vi "Setup For Triggered Images USB3 v4.3.vi"(5 "error in":errorcluster caption="error in (no error)", 6 "Timeout":u32, 7 "Gain":dbl, 8 "Shutter speed":dbl=0.1, 9 "Camera Name":T3="cam0") -> (0 "Error out":errorcluster caption="error in (no error)", 1 "Session Out":T3="cam0", 2 "Height":u32, 3 "Width":u32, 4 "DeviceID":string)   [LabVIEW 2013]
doc: "The Grab and Attributes Setup VI acquires images continuously and displays the images in an image control using high-level acquisition VIs. The VI also modifes the camera attributes while acquiring images. A grab is appropriate for high-speed applications in which you need to process only one image at a time."
uses:
  <vilib>/userdefined/High Color/IMAQdx.ctl
  <vilib>/vision/driver/IMAQdx.llb/IMAQdx Attribute Type.ctl
  <vilib>/vision/driver/IMAQdx.llb/IMAQdx Attribute Visibility.ctl
  <vilib>/vision/driver/NI_Vision_Acquisition_Software.lvlib
  <resource>/objmgr/imaqdx.rc
panel:
  out "Attribute Information Array":T2(array[cluster])=[{"Attribute Type"=enum."DBL", "Readable"=TRUE, "Writable"=TRUE, "Attribute Name"="CameraAttributes::AnalogControl::Gain"}, {"Attribute Type"=enum."DBL", "Readable"=TRUE, "Writable"=TRUE, "Attribute Name"="CameraAttributes::AnalogControl::BlackLevel"}, {"Attribute Type"=enum."DBL", "Readable"=TRUE, "Writable"=FALSE, "Attribute Name"="CameraAttributes::AnalogControl::Gamma"}, {"Attribute Type"=enum."Bool", "Readable"=TRUE, "Writable"=TRUE, "Attribute Name"="CameraAttributes::AnalogControl::GammaEnabled"}, {"Attribute Type"=enum."I64", "Readable"=TRUE, "Writable"=FALSE, "Attribute Name"="CameraAttributes::AnalogControl::Sharpness"}, {"Attribute Type"=enum."String", "Readable"=TRUE, "Writable"=FALSE, "Attribute Name"="CameraAttributes::DeviceControl::DeviceVendorName"}, {"Attribute Type"=enum."String", "Readable"=TRUE, "Writable"=FALSE, "Attribute Name"="CameraAttributes::DeviceControl::DeviceModelName"}, {"Attribute Type"=enum."String", "Readable"=TRUE, "Writable"=FALSE, "Attribute Name"="CameraAttributes::DeviceControl::DeviceFamilyName"}, {"Attribute Type"=enum."String", "Readable"=TRUE, "Writable"=FALSE, "Attribute Name"="CameraAttributes::DeviceControl::DeviceVersion"}, {"Attribute Type"=enum."String", "Readable"=TRUE, "Writable"=FALSE, "Attribute Name"="CameraAttributes::DeviceControl::DeviceSVNVersion"}, {"Attribute Type"=enum."String", "Readable"=TRUE, "Writable"=FALSE, "Attribute Name"="CameraAttributes::DeviceControl::DeviceID"}, {"Attribute Type"=enum."String", "Readable"=TRUE, "Writable"=TRUE, "Attribute Name"="CameraAttributes::DeviceControl::DeviceUserID"}, {"Attribute Type"=enum."Enum", "Readable"=TRUE, "Writable"=TRUE, "Attribute Name"="CameraAttributes::AcquisitionControl::TriggerSelector"}, {"Attribute Type"=enum."Enum", "Readable"=TRUE, "Writable"=TRUE, "Attribute Name"="CameraAttributes::AcquisitionControl::TriggerMode"}, {"Attribute Type"=enum."Command", "Readable"=FALSE, "Writable"=FALSE, "Attribute Name"="CameraAttributes::AcquisitionControl::TriggerSoftware"}, {"Attribute Type"=enum."Enum", "Readable"=TRUE, "Writable"=TRUE, "Attribute Name"="CameraAttributes::AcquisitionControl::TriggerSource"}, {"Attribute Type"=enum."Enum", "Readable"=TRUE, "Writable"=TRUE, "Attribute Name"="CameraAttributes::AcquisitionControl::TriggerActivation"}, {"Attribute Type"=enum."Enum", "Readable"=TRUE, "Writable"=TRUE, "Attribute Name"="CameraAttributes::AcquisitionControl::ExposureMode"}, {"Attribute Type"=enum."Enum", "Readable"=FALSE, "Writable"=FALSE, "Attribute Name"="CameraAttributes::AcquisitionControl::ExposureAuto"}, {"Attribute Type"=enum."DBL", "Readable"=TRUE, "Writable"=FALSE, "Attribute Name"="CameraAttributes::AcquisitionControl::ExposureTime"}, {"Attribute Type"=enum."Enum", "Readable"=TRUE, "Writable"=TRUE, "Attribute Name"="CameraAttributes::AcquisitionControl::AcquisitionMode"}, {"Attribute Type"=enum."Enum", "Readable"=TRUE, "Writable"=FALSE, "Attribute Name"="CameraAttributes::AcquisitionControl::AcquisitionFrameRateAuto"}, {"Attribute Type"=enum."Bool", "Readable"=FALSE, "Writable"=FALSE, "Attribute Name"="CameraAttributes::AcquisitionControl::AcquisitionFrameRateEnabled"}, {"Attribute Type"=enum."DBL", "Readable"=FALSE, "Writable"=FALSE, "Attribute Name"="CameraAttributes::AcquisitionControl::AcquisitionFrameRate"}, {"Attribute Type"=enum."I64", "Readable"=FALSE, "Writable"=FALSE, "Attribute Name"="CameraAttributes::AcquisitionControl::AcquisitionFrameCount"}, {"Attribute Type"=enum."Enum", "Readable"=TRUE, "Writable"=TRUE, "Attribute Name"="CameraAttributes::ImageFormatControl::PixelFormat"}, {"Attribute Type"=enum."I64", "Readable"=TRUE, "Writable"=TRUE, "Attribute Name"="CameraAttributes::ImageFormatControl::Width"}, {"Attribute Type"=enum."I64", "Readable"=TRUE, "Writable"=TRUE, "Attribute Name"="CameraAttributes::ImageFormatControl::Height"}, {"Attribute Type"=enum."I64", "Readable"=TRUE, "Writable"=TRUE, "Attribute Name"="CameraAttributes::ImageFormatControl::OffsetX"}, {"Attribute Type"=enum."I64", "Readable"=TRUE, "Writable"=TRUE, "Attribute Name"="CameraAttributes::ImageFormatControl::OffsetY"}, {"Attribute Type"=enum."Enum", "Readable"=TRUE, "Writable"=FALSE, "Attribute Name"="CameraAttributes::ImageFormatControl::PixelCoding"}, {"Attribute Type"=enum."I64", "Readable"=TRUE, "Writable"=FALSE, "Attribute Name"="CameraAttributes::ImageFormatControl::PixelDynamicRangeMin"}, {"Attribute Type"=enum."I64", "Readable"=TRUE, "Writable"=FALSE, "Attribute Name"="CameraAttributes::ImageFormatControl::PixelDynamicRangeMax"}, {"Attribute Type"=enum."Enum", "Readable"=TRUE, "Writable"=TRUE, "Attribute Name"="CameraAttributes::ImageFormatControl::TestImageSelector"}, {"Attribute Type"=enum."I64", "Readable"=TRUE, "Writable"=FALSE, "Attribute Name"="CameraAttributes::UserSetControl::UserSetCurrent"}, {"Attribute Type"=enum."Enum", "Readable"=TRUE, "Writable"=TRUE, "Attribute Name"="CameraAttributes::UserSetControl::UserSetSelector"}, {"Attribute Type"=enum."Command", "Readable"=FALSE, "Writable"=TRUE, "Attribute Name"="CameraAttributes::UserSetControl::UserSetLoad"}, {"Attribute Type"=enum."Command", "Readable"=FALSE, "Writable"=TRUE, "Attribute Name"="CameraAttributes::UserSetControl::UserSetSave"}, {"Attribute Type"=enum."DBL", "Readable"=FALSE, "Writable"=FALSE, "Attribute Name"="CameraAttributes::DigitalIOControl::StrobeDelay"}, {"Attribute Type"=enum."DBL", "Readable"=FALSE, "Writable"=FALSE, "Attribute Name"="CameraAttributes::DigitalIOControl::StrobeDuration"}]
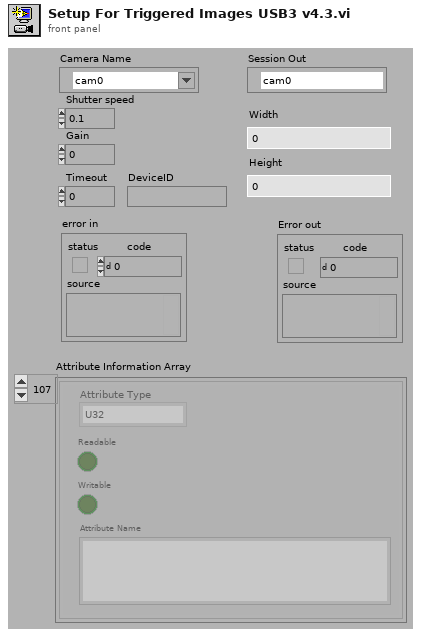
[diagram p1: front panel]
types:
  T1 = typedef "NI_Vision_Acquisition_Software.lvlib/IMAQdx Attribute Type.ctl" = enum32{"U32", "I64", "DBL", "String", "Enum", "Bool", "Command"}
  T2 = cluster{"Attribute Type":T1, "Readable":bool, "Writable":bool, "Attribute Name":string}[]
  T3 = typedef "IMAQdx.ctl" = refnum<k21>
  T4 = typedef "NI_Vision_Acquisition_Software.lvlib/IMAQdx Attribute Visibility.ctl" = enum32{"Simple", "Intermediate", "Advanced"}
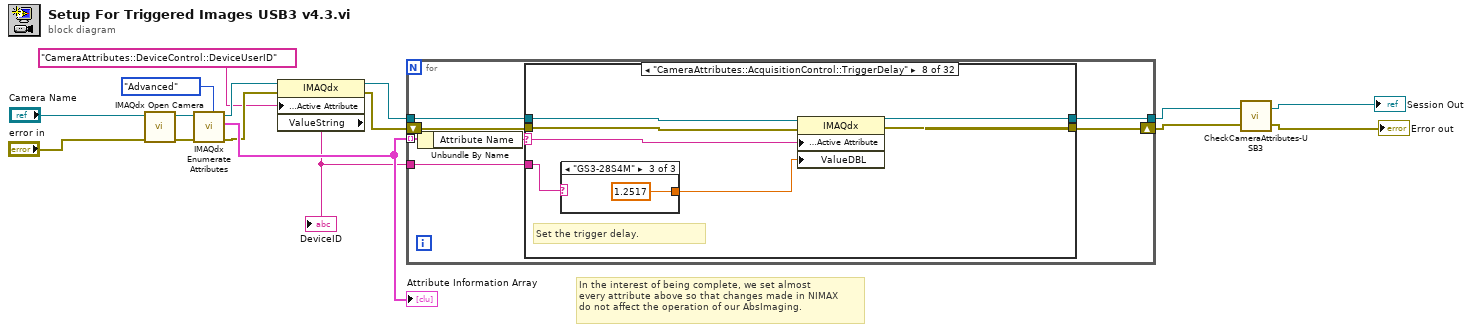
[diagram p0: block diagram]
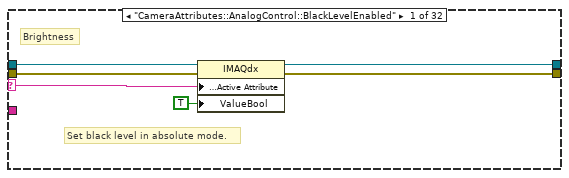
[diagram p2: hidden frame]
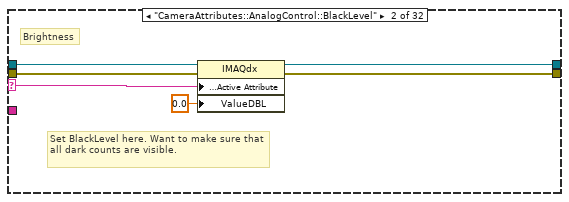
[diagram p3: hidden frame]
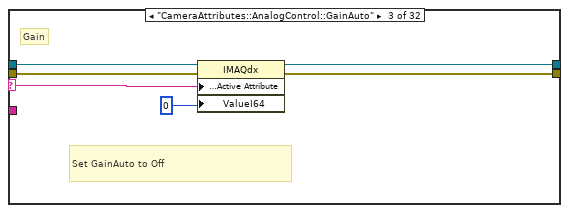
[diagram p4: hidden frame]
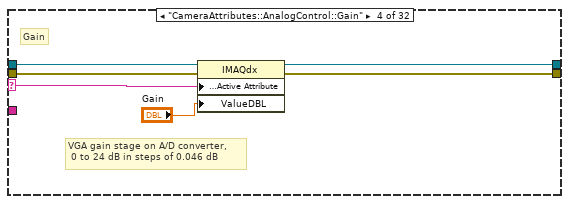
[diagram p5: hidden frame]
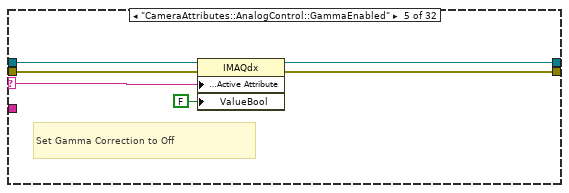
[diagram p6: hidden frame]
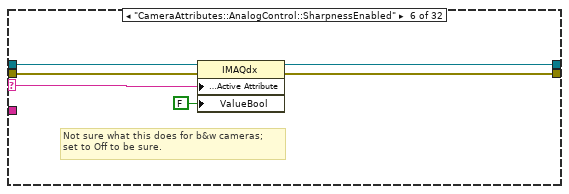
[diagram p7: hidden frame]
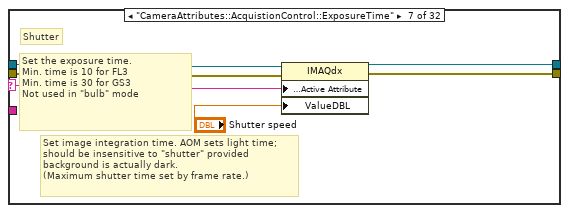
[diagram p8: hidden frame]
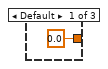
[diagram p9: hidden frame]
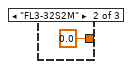
[diagram p10: hidden frame]
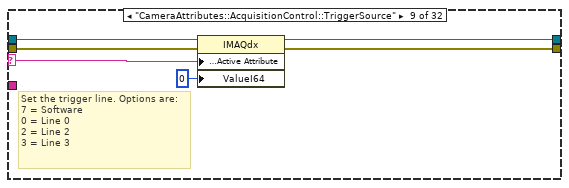
[diagram p11: hidden frame]
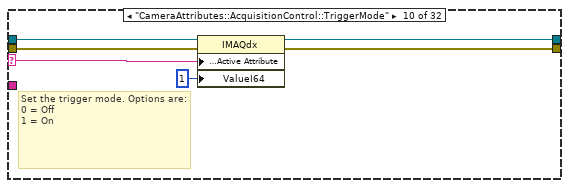
[diagram p12: hidden frame]
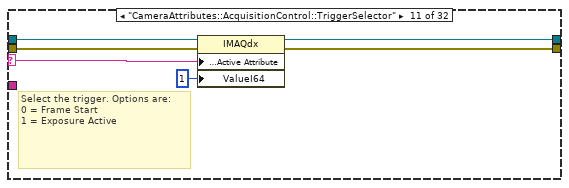
[diagram p13: hidden frame]
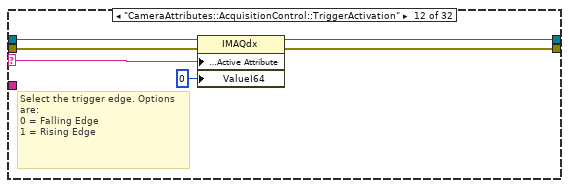
[diagram p14: hidden frame]
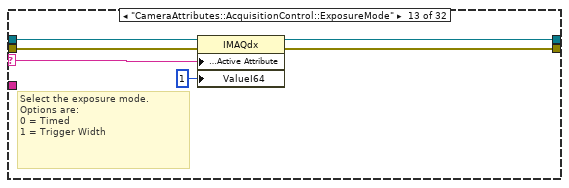
[diagram p15: hidden frame]
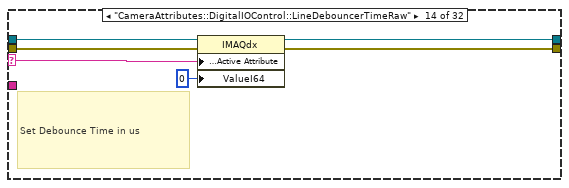
[diagram p16: hidden frame]
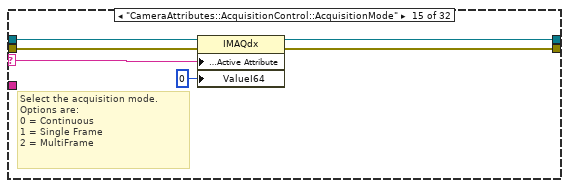
[diagram p17: hidden frame]
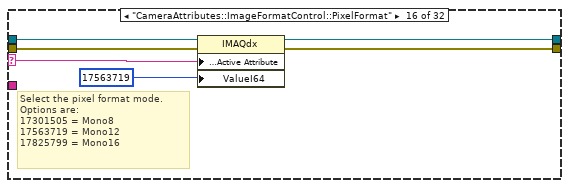
[diagram p18: hidden frame]
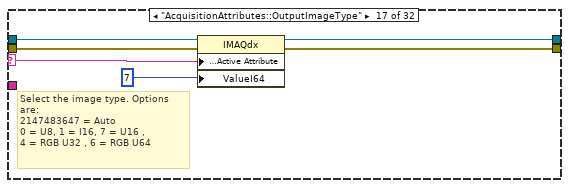
[diagram p19: hidden frame]
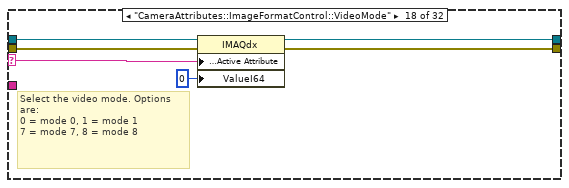
[diagram p20: hidden frame]
diagram:
  # "In the interest of being complete, we set almost\nevery attribute above so that changes made in NIMAX\ndo not affect the operation of our AbsImaging."
  n1 = call <vilib>:"IMAQdx Open Camera.vi"("error in"="error in", "Session In"="Camera Name") -> ("error out"=w14:errorcluster, "Session Out"=w15:T3)  [unwired: 1 in, 7 out]
  n2 = call <vilib>:"IMAQdx Enumerate Attributes.vi"("Visibility"=IMAQdx_Attribute_Visibility."Advanced", "error in"=w14, "Session In"=w15) -> ("error out"=w9:errorcluster, "Attribute Information Array"=w11:T2, "Session Out"=w10:T3)  [unwired: 1 in, 5 out]
  "Attribute Information Array" <- w11
  n3 = property class="IMAQdx"(reference=w10, error in=w9, "Camera Attributes:Active Attribute"="CameraAttributes::DeviceControl::DeviceUserID" ("ActiveAttribute")) -> (reference out=w7:T3, error out=w8:errorcluster, "ValueString"=w6:string)
  "DeviceID" <- w6
  n4 = for {
    tunnel: w11 -> [w23] mode=indexing
    tunnel: w7 -> [w18]
    tunnel: [w21] -> w3
    shift-right: [w20] -> w4
    shift-left: w8 -> [w19]
    tunnel: w6 -> [w17]
    n5 = Unbundle By Name(w23) -> ("Attribute Name"=w22:string)
    n6 = case shown="\"CameraAttributes::AcquisitionControl::TriggerDelay\"" w22 {
      selector: w22 -> [w25 w31 w37 w43 w49 w55 w61 w68 w77 w83 w89 w95 w101 w107 w113 w119 w125 w131 w137 w143 w151 w161 w170 w176 w182 w188 w194 w199 w205 w211 w217 _]
      tunnel: w18 -> [w29 w35 w41 w47 w53 w59 w65 w72 w81 w87 w93 w99 w105 w111 w117 w123 w129 w135 w141 w147 w150 w160 w169 w175 w181 w187 w193 w203 w209 w215 w221 w223]
      tunnel: w19 -> [w28 w34 w40 w46 w52 w58 w64 w71 w80 w86 w92 w98 w104 w110 w116 w122 w128 w134 w140 w146 w154 w164 w173 w179 w185 w191 w197 w202 w208 w214 w220 w222]
      tunnel: [w27 w33 w39 w45 w51 w57 w63 w70 w79 w85 w91 w97 w103 w109 w115 w121 w127 w133 w139 w145 w153 w163 w172 w178 w184 w190 w196 w201 w207 w213 w219 w223] -> w21
      tunnel: [w26 w32 w38 w44 w50 w56 w62 w69 w78 w84 w90 w96 w102 w108 w114 w120 w126 w132 w138 w144 w152 w162 w171 w177 w183 w189 w195 w200 w206 w212 w218 w222] -> w20
      tunnel: w17 -> [_ _ _ _ _ _ _ w67 _ _ _ _ _ _ _ _ _ _ _ _ w149 w159 _ _ _ _ _ _ _ _ _ _]
      frame "CameraAttributes::AnalogControl::BlackLevelEnabled" {
        # "Set black level in absolute mode."
        # "Brightness"
        n7 = property class="IMAQdx"(reference=w29, error in=w28, "Camera Attributes:Active Attribute"=w25, "ValueBool"=TRUE) -> (reference out=w27:T3, error out=w26:errorcluster)
      }
      frame "CameraAttributes::AnalogControl::BlackLevel" {
        # "Set BlackLevel here. Want to make sure that all dark counts are visible."
        # "Brightness"
        n8 = property class="IMAQdx"(reference=w35, error in=w34, "Camera Attributes:Active Attribute"=w31, "ValueDBL"=0.0) -> (reference out=w33:T3, error out=w32:errorcluster)
      }
      frame "CameraAttributes::AnalogControl::GainAuto" {
        # "Set GainAuto to Off"
        # "Gain"
        n9 = property class="IMAQdx"(reference=w41, error in=w40, "Camera Attributes:Active Attribute"=w37, "ValueI64"=i64 0) -> (reference out=w39:T3, error out=w38:errorcluster)
      }
      frame "CameraAttributes::AnalogControl::Gain" {
        # "VGA gain stage on A/D converter,\n 0 to 24 dB in steps of 0.046 dB"
        # "Gain"
        n10 = property class="IMAQdx"(reference=w47, error in=w46, "Camera Attributes:Active Attribute"=w43, "ValueDBL"="Gain") -> (reference out=w45:T3, error out=w44:errorcluster)
      }
      frame "CameraAttributes::AnalogControl::GammaEnabled" {
        # "Set Gamma Correction to Off"
        n11 = property class="IMAQdx"(reference=w53, error in=w52, "Camera Attributes:Active Attribute"=w49, "ValueBool"=FALSE) -> (reference out=w51:T3, error out=w50:errorcluster)
      }
      frame "CameraAttributes::AnalogControl::SharpnessEnabled" {
        # "Not sure what this does for b&w cameras;\nset to Off to be sure."
        n12 = property class="IMAQdx"(reference=w59, error in=w58, "Camera Attributes:Active Attribute"=w55, "ValueBool"=FALSE) -> (reference out=w57:T3, error out=w56:errorcluster)
      }
      frame "CameraAttributes::AcquistionControl::ExposureTime" {
        # "Set the exposure time.\nMin. time is 10 for FL3\nMin. time is 30 for GS3\nNot used in \"bulb\" mode"
        # "Set image integration time. AOM sets light time;\nshould be insensitive to \"shutter\" provided \nbackground is actually dark.\n(Maximum shutter time set by frame rate.)"
        # "Shutter"
        n13 = property class="IMAQdx"(reference=w65, error in=w64, "Camera Attributes:Active Attribute"=w61, "ValueDBL"="Shutter speed") -> (reference out=w63:T3, error out=w62:errorcluster)
      }
      frame "CameraAttributes::AcquisitionControl::TriggerDelay" {
        # "Set the trigger delay."
        n14 = case shown="\"GS3-28S4M\"" w67 {
          tunnel: [0.0 ("ValueDBL") 0.0 ("ValueDBL") 1.2517 ("ValueDBL")] -> w66
          frame Default {
          }
          frame "FL3-32S2M" {
          }
          frame "GS3-28S4M" {
          }
        }
        n15 = property class="IMAQdx"(reference=w72, error in=w71, "Camera Attributes:Active Attribute"=w68, "ValueDBL"=w66) -> (reference out=w70:T3, error out=w69:errorcluster)
      }
      frame "CameraAttributes::AcquisitionControl::TriggerSource" {
        # "Set the trigger line. Options are:\n7 = Software\n0 = Line 0\n2 = Line 2\n3 = Line 3"
        n16 = property class="IMAQdx"(reference=w81, error in=w80, "Camera Attributes:Active Attribute"=w77, "ValueI64"=i64 0) -> (reference out=w79:T3, error out=w78:errorcluster)
      }
      frame "CameraAttributes::AcquisitionControl::TriggerMode" {
        # "Set the trigger mode. Options are:\n0 = Off\n1 = On"
        n17 = property class="IMAQdx"(reference=w87, error in=w86, "Camera Attributes:Active Attribute"=w83, "ValueI64"=i64 1) -> (reference out=w85:T3, error out=w84:errorcluster)
      }
      frame "CameraAttributes::AcquisitionControl::TriggerSelector" {
        # "Select the trigger. Options are:\n0 = Frame Start\n1 = Exposure Active"
        n18 = property class="IMAQdx"(reference=w93, error in=w92, "Camera Attributes:Active Attribute"=w89, "ValueI64"=i64 1) -> (reference out=w91:T3, error out=w90:errorcluster)
      }
      frame "CameraAttributes::AcquisitionControl::TriggerActivation" {
        # "Select the trigger edge. Options are:\n0 = Falling Edge\n1 = Rising Edge"
        n19 = property class="IMAQdx"(reference=w99, error in=w98, "Camera Attributes:Active Attribute"=w95, "ValueI64"=i64 0) -> (reference out=w97:T3, error out=w96:errorcluster)
      }
      frame "CameraAttributes::AcquisitionControl::ExposureMode" {
        # "Select the exposure mode. Options are:\n0 = Timed\n1 = Trigger Width"
        n20 = property class="IMAQdx"(reference=w105, error in=w104, "Camera Attributes:Active Attribute"=w101, "ValueI64"=i64 1) -> (reference out=w103:T3, error out=w102:errorcluster)
      }
      frame "CameraAttributes::DigitalIOControl::LineDebouncerTimeRaw" {
        # "Set Debounce Time in us"
        n21 = property class="IMAQdx"(reference=w111, error in=w110, "Camera Attributes:Active Attribute"=w107, "ValueI64"=i64 0) -> (reference out=w109:T3, error out=w108:errorcluster)
      }
      frame "CameraAttributes::AcquisitionControl::AcquisitionMode" {
        # "Select the acquisition mode. Options are:\n0 = Continuous\n1 = Single Frame\n2 = MultiFrame"
        n22 = property class="IMAQdx"(reference=w117, error in=w116, "Camera Attributes:Active Attribute"=w113, "ValueI64"=i64 0) -> (reference out=w115:T3, error out=w114:errorcluster)
      }
      frame "CameraAttributes::ImageFormatControl::PixelFormat" {
        # "Select the pixel format mode. Options are:\n17301505 = Mono8\n17563719 = Mono12\n17825799 = Mono16"
        n23 = property class="IMAQdx"(reference=w123, error in=w122, "Camera Attributes:Active Attribute"=w119, "ValueI64"=i64 17563719) -> (reference out=w121:T3, error out=w120:errorcluster)
      }
      frame "AcquisitionAttributes::OutputImageType" {
        # "Select the image type. Options are:\n2147483647 = Auto\n0 = U8, 1 = I16, 7 = U16 , \n4 = RGB U32 , 6 = RGB U64"
        n24 = property class="IMAQdx"(reference=w129, error in=w128, "Camera Attributes:Active Attribute"=w125, "ValueI64"=i64 7) -> (reference out=w127:T3, error out=w126:errorcluster)
      }
      frame "CameraAttributes::ImageFormatControl::VideoMode" {
        # "Select the video mode. Options are:\n0 = mode 0, 1 = mode 1\n7 = mode 7, 8 = mode 8"
        n25 = property class="IMAQdx"(reference=w135, error in=w134, "Camera Attributes:Active Attribute"=w131, "ValueI64"=i64 0) -> (reference out=w133:T3, error out=w132:errorcluster)
      }
      frame "CameraAttributes::AcquisitionControl::pgrExposureCompensationAuto" {
        # "Select the exposure compensation mode. Options are:\n0 = off, 2 = continuous"
        n26 = property class="IMAQdx"(reference=w141, error in=w140, "Camera Attributes:Active Attribute"=w137, "ValueU32"=u32 0) -> (reference out=w139:T3, error out=w138:errorcluster)
      }
      frame "CameraAttributes::AcquisitionControl::pgrExposureCompensation" {
        # "Select the exposure compensation in EV\n\n0.001 gives zero"
        n27 = property class="IMAQdx"(reference=w147, error in=w146, "Camera Attributes:Active Attribute"=w143, "ValueDBL"=0.001) -> (reference out=w145:T3, error out=w144:errorcluster)
      }
      frame "CameraAttributes::ImageFormatControl::Width" {
        # "Select the width. Max is 2080 for FL3\nMax is 1928 for GH3"
        n28 = case shown="\"GS3-28S4M\"" w149 {
          tunnel: [i64 100 ("ValueI64") i64 2080 ("ValueI64") i64 1928 ("ValueI64")] -> w148
          frame Default {
          }
          frame "FL3-32S2M" {
          }
          frame "GS3-28S4M" {
          }
        }
        "Width" <- w148
        n29 = property class="IMAQdx"(reference=w150, error in=w154, "Camera Attributes:Active Attribute"=w151, "ValueI64"=w148) -> (reference out=w153:T3, error out=w152:errorcluster)
      }
      frame "CameraAttributes::ImageFormatControl::Height" {
        # "Select the height. Max is 1552 for FL3\nMax is 1448 for GH3"
        n30 = case shown="\"GS3-28S4M\"" w159 {
          tunnel: [i64 100 ("ValueI64") i64 1552 ("ValueI64") i64 1448 ("ValueI64")] -> w158
          frame Default {
          }
          frame "FL3-32S2M" {
          }
          frame "GS3-28S4M" {
          }
        }
        "Height" <- w158
        n31 = property class="IMAQdx"(reference=w160, error in=w164, "Camera Attributes:Active Attribute"=w161, "ValueI64"=w158) -> (reference out=w163:T3, error out=w162:errorcluster)
      }
      frame "CameraAttributes::ImageFormatControl::OffsetX" {
        # "Select the X offset."
        n32 = property class="IMAQdx"(reference=w169, error in=w173, "Camera Attributes:Active Attribute"=w170, "ValueI64"=i64 0) -> (reference out=w172:T3, error out=w171:errorcluster)
      }
      frame "CameraAttributes::ImageFormatControl::OffsetY" {
        # "Select the Y offset."
        n33 = property class="IMAQdx"(reference=w175, error in=w179, "Camera Attributes:Active Attribute"=w176, "ValueI64"=i64 0) -> (reference out=w178:T3, error out=w177:errorcluster)
      }
      frame "CameraAttributes::ImageFormatControl::BinningVertical" {
        # "No vertical binning"
        n34 = property class="IMAQdx"(reference=w181, error in=w185, "Camera Attributes:Active Attribute"=w182, "ValueI64"=i64 1) -> (reference out=w184:T3, error out=w183:errorcluster)
      }
      frame "AcquisitionAttributes::Timeout" {
        # "Set the timeout"
        n35 = property class="IMAQdx"(reference=w187, error in=w191, "Camera Attributes:Active Attribute"=w188, "ValueU32"="Timeout") -> (reference out=w190:T3, error out=w189:errorcluster)
      }
      frame "CameraAttributes::ImageFormatControl::ReverseX" {
        # "Reverse X or not"
        n36 = property class="IMAQdx"(reference=w193, error in=w197, "Camera Attributes:Active Attribute"=w194, "ValueBool"=FALSE) -> (reference out=w196:T3, error out=w195:errorcluster)
      }
      frame "CameraAttributes::AcquisitionControl::TriggerDelayEnabled" {
        # "Do not want any TriggerDelay"
        n37 = property class="IMAQdx"(reference=w203, error in=w202, "Camera Attributes:Active Attribute"=w199, "ValueBool"=FALSE) -> (reference out=w201:T3, error out=w200:errorcluster)
      }
      frame "AcquisitionAttributes::SwapPixelBytes" {
        # "Don't swap bytes"
        n38 = property class="IMAQdx"(reference=w209, error in=w208, "Camera Attributes:Active Attribute"=w205, "ValueBool"=FALSE) -> (reference out=w207:T3, error out=w206:errorcluster)
      }
      frame "AcquisitionAttributes::ShiftPixelBits" {
        # "Don't shift bits"
        n39 = property class="IMAQdx"(reference=w215, error in=w214, "Camera Attributes:Active Attribute"=w211, "ValueBool"=FALSE) -> (reference out=w213:T3, error out=w212:errorcluster)
      }
      frame "CameraAttributes::ImageFormatControl::PixelDefectControl::pgrDefectPixelCorrectionEnable" {
        # "Turn on defect control"
        n40 = property class="IMAQdx"(reference=w221, error in=w220, "Camera Attributes:Active Attribute"=w217, "ValueBool"=TRUE) -> (reference out=w219:T3, error out=w218:errorcluster)
      }
      frame Default {
      }
    }
  }
  n41 = call "CheckCameraAttributes-USB3.vi"("error in"=w4, "Camera Name"=w3) -> ("error out"=→"Error out":errorcluster, "Session Out"=→"Session Out":T3)
